vi "Get Lockstep Info.vi"(8 "error in (no error)":errorcluster, 9 "Device Number":string, 10 "Lockstep Group (1)":u8=1, 11 "VISA resource name":refnum<visa-resource-name>) -> (0 "error out":errorcluster, 1 "Axis Offsets":i32[](array[numeric]), 2 "Axis Numbers":i32[](array[numeric]), 3 "VISA resource name out":refnum<visa-resource-name>, 4 "Axis Twists":i32[](array[numeric]))   [LabVIEW 2013, in "Zaber A Series.lvlib"]
doc: "Returns information about a lockstep group. The outputs are:\n- The axis numbers of the axes in the group.\n- The position offsets of each axis relative to the first one, in microsteps.\n- The current twist of each axis relative to the first one.\n\nNote that at present only two axes per group are supported.\n\nThis VI requires that the Initialize VI has been called with the same serial port and that the specified lockstep group has been configured."
uses:
  Zaber A Series.lvlib
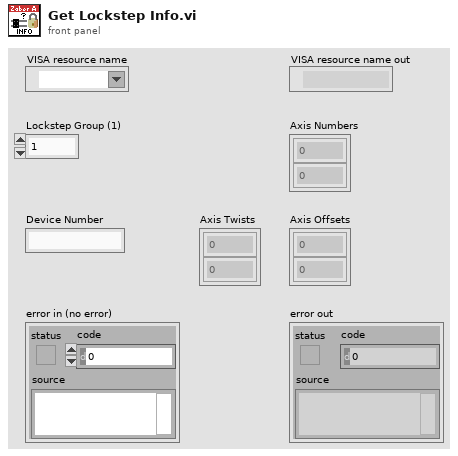
[diagram p1: front panel]
types:
  T1 = cluster{"Device":string, "Axis":string, "Reply Flag":string, "Status":string, "Warning Flags":string, "Data":string}
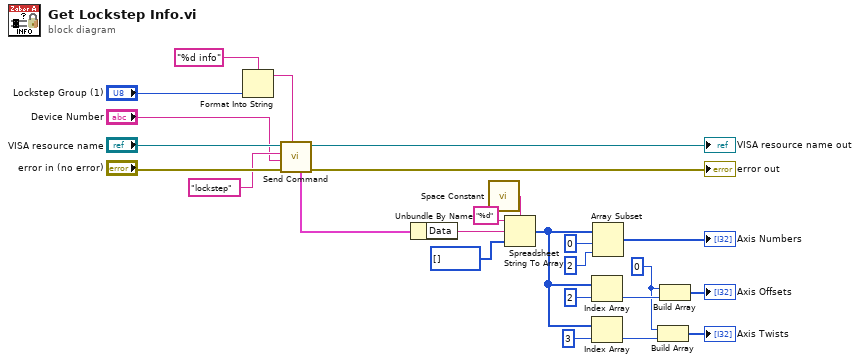
[diagram p0: block diagram]
diagram:
  w11 = 0 ("element")
  n1 = Format Into String(format string="%d info", "Lockstep Group (1)") -> (resulting string=w2:string)  [unwired: 2 in, 1 out]
  n2 = call "Send Command.vi"("Data"=w2, "error in (no error)"="error in (no error)", "Device and Axis"="Device Number", "Command"="lockstep", "VISA resource name"="VISA resource name") -> ("error out"=→"error out":errorcluster, "VISA resource name out"=→"VISA resource name out":refnum<visa-resource-name>, "First Response Bundle"=w1:T1)  [unwired: 1 in, 3 out]
  n3 = Unbundle By Name(w1) -> ("Data"=w22:string)
  n4 = call <vilib>:"Space Constant.vi"() -> ("String"=w23:string)
  n5 = Spreadsheet String To Array(delimiter (Tab)=w23, format string="%d", spreadsheet string=w22, array type (2D Dbl)=i32[] []) -> (array=w17:i32[])
  n6 = Index Array(array=w17, index=2) -> (element=w13:i32)
  n7 = Index Array(array=w17, index=3) -> (element=w10:i32)
  n8 = Array Subset(array=w17, index=0, length=2) -> (→"Axis Numbers":i32[])
  n9 = Build Array(w11, w10) -> (→"Axis Twists":i32[])
  n10 = Build Array(w11, w13) -> (→"Axis Offsets":i32[])
